vi "Example Graph.vi"() -> ()   [LabVIEW 2013]
uses:
  C:/tf/play/labview/Tinkerforge.dll
panel:
  in  "stop":bool
  out "graph":i32[](graph)
  in  "uid":string="8e7"
  in  "port":i32=4223
  in  "host":string="localhost"
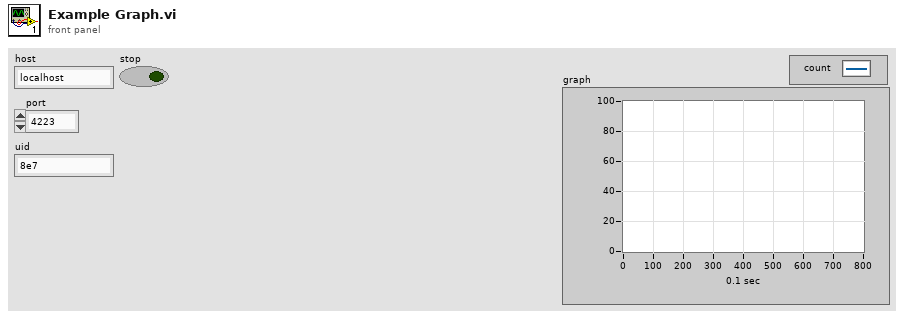
[diagram p1: front panel]
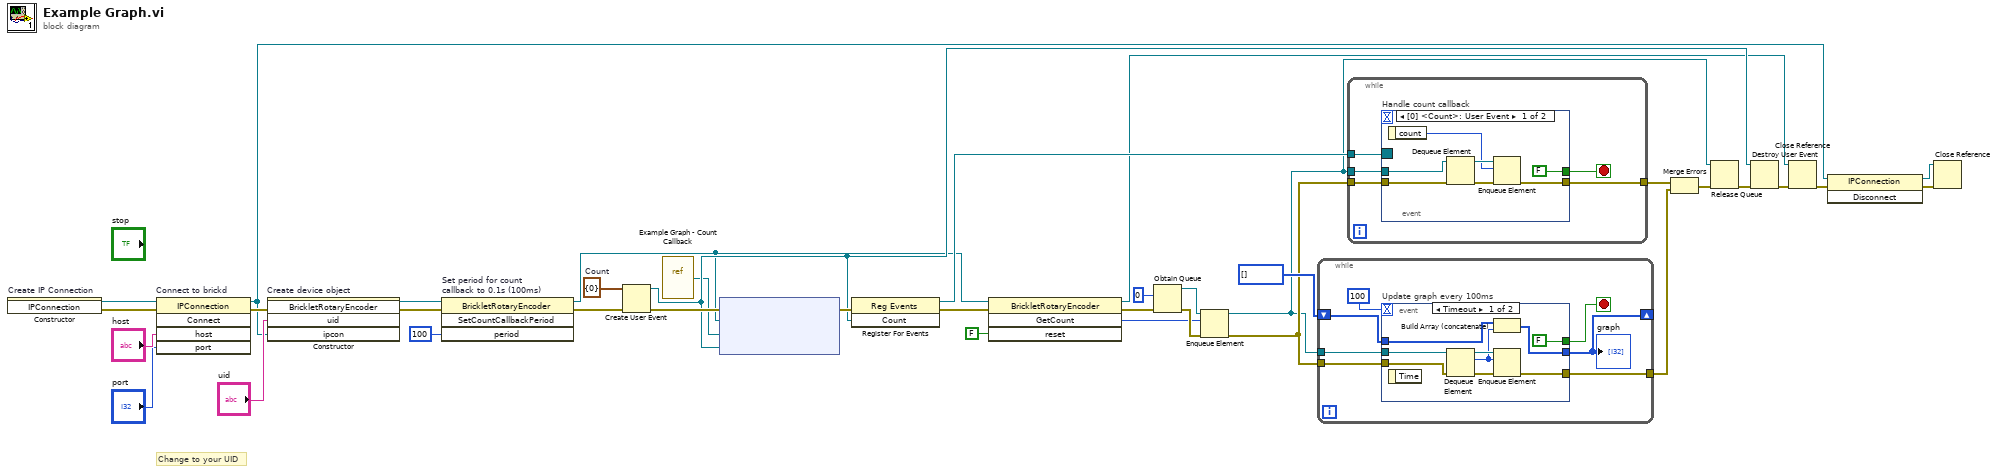
[diagram p0: block diagram]
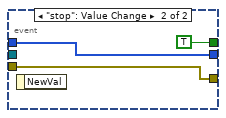
[diagram p2: hidden frame]
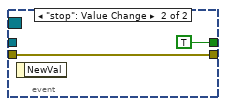
[diagram p3: hidden frame]
diagram:
  w23 = cluster{"count":i32} {"count"=0}  # Count
  # "Change to your UID"
  n1 = constructor on="Create IP Connection" class="IPConnection"() -> (reference out=w37:refnum<k24>, error out=w8:errorcluster)  [unwired: 3 in, 1 out]
  n2 = invoke on="Connect to brickd" class="IPConnection" method="Connect"(reference=w37, error in=w8, "host"="host", "port"="port") -> (reference out=w30:refnum<k24>, error out=w33:errorcluster)  [unwired: 1 in, 3 out]
  n3 = constructor on="Create device object" class="BrickletRotaryEncoder"(error in=w33, "uid"="uid", "ipcon"=w30) -> (reference out=w20:refnum<k24>, error out=w22:errorcluster)  [unwired: 2 in, 3 out]
  n4 = invoke on="Set period for count\ncallback to 0.1s (100ms)" class="BrickletRotaryEncoder" method="SetCountCallbackPeriod"(reference=w20, error in=w22, "period"=i64 100) -> (reference out=w5:refnum<k24>, error out=w21:errorcluster)  [unwired: 1 in, 2 out]
  n5 = Create User Event(user event datatype=w23, error in=w21) -> (user event=w25:refnum<user-event>, error out=w28:errorcluster)
  n6 = vi-ref "Example Graph - Count Callback.vi"() -> ("vi reference"=w2:refnum<vi>)
  n7 = node ("Register Event Callback")(w28, w5, w2, w25) -> (w27:errorcluster)  [unwired: 1 in, 1 out]
  n8 = register-events(error in=w27, w25) -> (reference out=w26:refnum<event-registration>, error out=w7:errorcluster)  [unwired: 1 in]
  n9 = invoke class="BrickletRotaryEncoder" method="GetCount"(reference=w5, error in=w7, "reset"=FALSE) -> (reference out=w4:refnum<k24>, error out=w6:errorcluster, "GetCount"=w3:i32)  [unwired: 1 in, 1 out]
  n10 = Obtain Queue(element data type=0, error in (no error)=w6) -> (queue out=w12:refnum<queue>, error out=w14:errorcluster)  [unwired: 3 in, 1 out]
  n11 = Enqueue Element(queue=w12, element=w3, error in (no error)=w14) -> (queue out=w9:refnum<queue>, error out=w13:errorcluster)  [unwired: 1 in, 1 out]
  n12 = while {
    tunnel: [w40] -> w18
    tunnel: w13 -> [w41]
    shift-right: [w42] -> _
    shift-left: i32[] [] -> [w43]
    tunnel: w9 -> [w39]
    stop <- w38 stop-if-true
    n13 = event "Update graph every 100ms" shown="[0] Timeout" {
      selector: _ -> [_ _]
      dyn-events: _ -> [_ _]
      timeout: 100 -> [_ _]
      tunnel: [w53 w55] -> w42
      tunnel: w43 -> [w46 w55]
      tunnel: w41 -> [w52 w54]
      tunnel: [w49 w54] -> w40
      tunnel: w39 -> [w51 _]
      tunnel: [FALSE TRUE] -> w38
      event Timeout {
        n14 = event-data() -> ()  [unwired: 1 in, 1 out]
        n15 = Dequeue Element(queue=w51, error in (no error)=w52) -> (queue out=w48:refnum<queue>, element=w47:i32, error out=w50:errorcluster)  [unwired: 1 in, 1 out]
        n16 = Build Array (concatenate)(w46, w47) -> (w53:i32[])
        n17 = Enqueue Element(queue=w48, element=w47, error in (no error)=w50) -> (error out=w49:errorcluster)  [unwired: 1 in, 2 out]
      }
      event "stop": Value Change {
        n18 = event-data() -> ()  [unwired: 1 in, 1 out]
      }
    }
    "graph" <- w42
  }
  n19 = while {
    tunnel: w26 -> [w61]
    tunnel: [w59] -> w17
    tunnel: w13 -> [w60]
    tunnel: w9 -> [w58]
    stop <- w57 stop-if-true
    n20 = event "Handle count callback" shown="[0] <Count>: User Event" {
      selector: w61 -> [_ _]
      dyn-events: _ -> [_ _]
      timeout: _ -> [_ _]
      tunnel: w60 -> [w68 w69]
      tunnel: [w66 w69] -> w59
      tunnel: w58 -> [w65 _]
      tunnel: [FALSE TRUE] -> w57
      event User Event {
        n21 = event-data() -> ("count"=w62:i32)  [unwired: 1 in]
        n22 = Dequeue Element(queue=w65, error in (no error)=w68) -> (queue out=w64:refnum<queue>, error out=w67:errorcluster)  [unwired: 1 in, 2 out]
        n23 = Enqueue Element(queue=w64, element=w62, error in (no error)=w67) -> (error out=w66:errorcluster)  [unwired: 1 in, 2 out]
      }
      event "stop": Value Change {
        n24 = event-data() -> ()  [unwired: 1 in, 1 out]
      }
    }
  }
  n25 = Merge Errors(w17, w18) -> (w11:errorcluster)
  n26 = Release Queue(queue=w9, error in (no error)=w11) -> (error out=w10:errorcluster)  [unwired: 1 in, 2 out]
  n27 = Destroy User Event(user event=w25, error in=w10) -> (error out=w24:errorcluster)
  n28 = Close Reference(reference=w4, error in (no error)=w24) -> (error out=w32:errorcluster)
  n29 = invoke class="IPConnection" method="Disconnect"(reference=w30, error in=w32) -> (reference out=w29:refnum<k24>, error out=w31:errorcluster)  [unwired: 1 in, 1 out]
  n30 = Close Reference(reference=w29, error in (no error)=w31) -> ()  [unwired: 1 out]
